vi "Set Power.vi"(8 "error in (no error)":errorcluster, 9 "Power (mW)":dbl, 11 "Cobolt Laser in":refnum<class "Cobolt Laser.lvclass">) -> (0 "error out":errorcluster, 3 "Cobolt Laser out":refnum<class "Cobolt Laser.lvclass">)   [LabVIEW 2023, in "Cobolt Laser.lvlib" / "Cobolt Laser.lvclass"]
uses:
  Cobolt Laser.lvclass
  Cobolt Laser.lvclass/Cobolt Laser.ctl
  Laser/Laser.lvclass
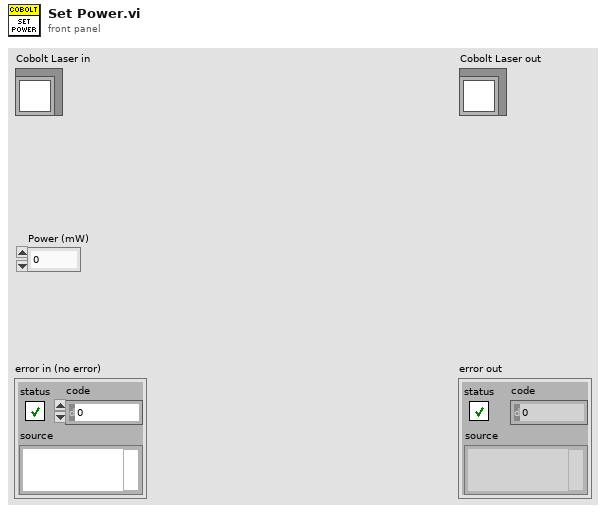
[diagram p1: front panel]
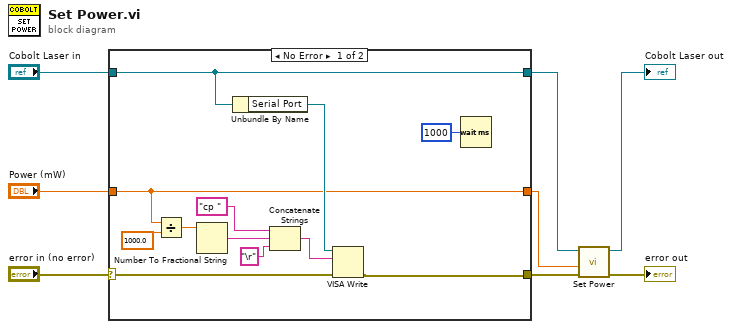
[diagram p0: block diagram]
diagram:
  n1 = case shown="No Error" "error in (no error)" {
    selector: "error in (no error)" -> [w20 w23]
    tunnel: [w13 w23] -> w5
    tunnel: "Cobolt Laser in" -> [w15 w22]
    tunnel: [w15 w22] -> w3
    tunnel: "Power (mW)" -> [w10 w21]
    tunnel: [w10 w21] -> w1
    frame No Error {
      n2 = Divide(x=w10, y=1000.0) -> (x/y=w11:dbl)
      n3 = Number To Fractional String(number=w11) -> (F-format string=w18:string)  [unwired: 3 in]
      n4 = Unbundle By Name(w15) -> ("Serial Port"=w14:refnum<visa-resource-name>)
      n5 = Concatenate Strings("cp " ("write buffer"), w18, "\r" ("string")) -> (w17:string)
      n6 = VISA Write(VISA resource name=w14, write buffer=w17, error in (no error)=w20) -> (error out=w13:errorcluster)  [unwired: 2 out]
      n7 = Wait (ms)(milliseconds to wait=u32 1000) -> ()  [unwired: 1 out]
    }
    frame Error {
    }
  }
  n8 = call-parent "Set Power.vi"("error in (no error)"=w5, "Power"=w1, "Laser Quantum in"=w3) -> ("error out"=→"error out":errorcluster, "Laser Quantum out"=→"Cobolt Laser out":refnum<class "Cobolt Laser.lvclass">)  [unwired: 7 in]
